vi "Configure Read Timeout.vi"(0 "UART Driver in":refnum<class "UART Driver.lvclass">, 5 "UART Read Timeout (s)":dbl=10.0, 11 "error in":errorcluster) -> (4 "UART Driver out":refnum<class "UART Driver.lvclass">, 15 "error out":errorcluster)   [LabVIEW 2012, in "UART_Host_Driver.lvlib" / "UART Driver.lvclass"]
doc: "Configure the UART Read Data Timeout."
uses:
  UART Driver.lvclass
  UART Driver.lvclass/UART Driver.ctl
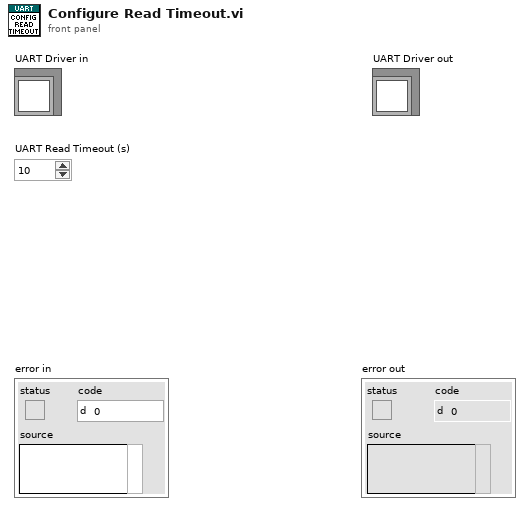
[diagram p1: front panel]
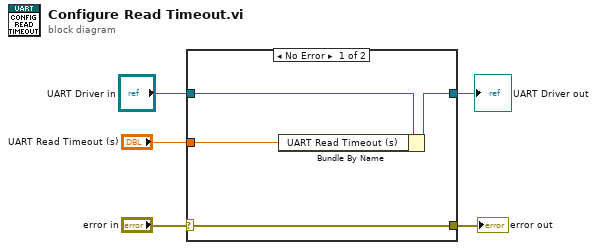
[diagram p0: block diagram]
diagram:
  n1 = case shown="No Error" "error in" {
    selector: "error in" -> [w9 w10]
    tunnel: [w9 w10] -> w4
    tunnel: [w7 w11] -> w2
    tunnel: "UART Driver in" -> [w8 w11]
    tunnel: "UART Read Timeout (s)" -> [w6 _]
    frame No Error {
      n2 = Bundle By Name(cluster=w8, "UART Read Timeout (s)"=w6) -> (w7:refnum<class "UART Driver.lvclass">)
    }
    frame Error {
    }
  }
  "error out" <- w4
  "UART Driver out" <- w2
